vi "Get Package Filters.vi"(7 "LabVIEW Web Service Request":refnum<class "Web Request.lvclass">) -> ()   [LabVIEW 2016]
uses:
  <vilib>/wsapi/Web Request.lvclass
  Repo_class/Repo.lvclass/Repo.ctl
  Package_class/Package.lvclass/Package.ctl
  Repo_class/Read Packages.vi
  Package_class/Read RepoType.vi
  Package_class/Read RepoName.vi
  WSsupport/GV_Repos.vi
  <userlib>/_OpenG.lib/array/array.llb/Remove Duplicates from 1D Array (String)__ogtk.vi
  <vilib>/addons/JSON API/Variant JSON/Variant to JSON.vi
  Package_class/Package.lvclass
  WSsupport/WSsupport.lvlib
  Repo_class/Repo.lvclass
  <vilib>/addons/JSON API/Get Polymorphic/JSON GetSet.lvlib
  <vilib>/addons/JSON API/JSON Value/JSON Value.lvclass
  ServerErrors/ServerErrors.lvlib
  <vilib>/addons/JSON API/Variant JSON/Variant JSON.lvlib
panel:
  # "Use the Web Service Request input terminal to call the VIs on the Web Services palette. Do not remove it from the connector pane unless you don't need access to the palette."
  # "Each additional control wired to the connector pane will be available as an input in the URL. To include an indicator in terminal-mode output (the default setting), it must also be wired to the connector pane."
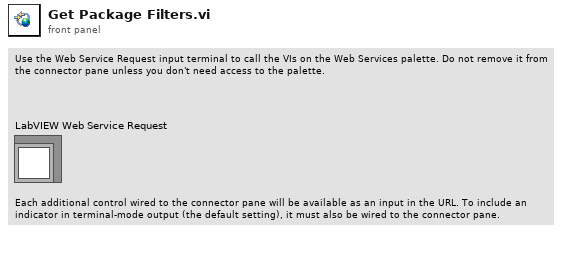
[diagram p1: front panel]
types:
  T1 = cluster{"RepoTypes":string[], "RepoNames":string[]}
  T2 = typedef "Packages.lvlib/Repo.lvclass/RepoType--enum.ctl" = enum16{"VIPM", "NIPM", "GPM"}
  T3 = typedef "ServerErrors.lvlib/Error Message--cluster.ctl" = cluster{"HTTP Code":i32, "JSON Response":cluster{"error":string, "reason":string}}
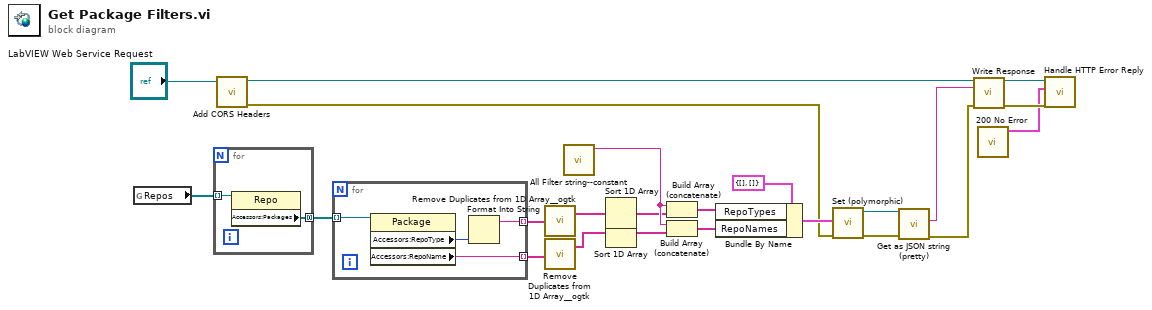
[diagram p0: block diagram]
diagram:
  n1 = global read "GV_Repos.vi" "Repos"() -> (w22:refnum<class "Repo.lvclass">[])
  n2 = for {
    tunnel: w22 -> [w25] mode=indexing
    tunnel: [w24] -> w21 mode=concatenating
    n3 = property class="Repo"(reference=w25) -> ("Accessors:Packages"=w24:refnum<class "Package.lvclass">[])  [unwired: 1 in, 2 out]
  }
  n4 = call "Add CORS Headers.vi"("LabVIEW Web Service Request"="LabVIEW Web Service Request") -> ("error out"=w12:errorcluster, "LabVIEW Web Service Request out"=w8:refnum<class "Web Request.lvclass">)  [unwired: 9 in]
  n5 = for {
    tunnel: w21 -> [w29] mode=indexing
    tunnel: [w27] -> w20 mode=indexing
    tunnel: [w26] -> w19 mode=indexing
    n6 = property class="Package"(reference=w29) -> ("Accessors:RepoType"=w28:T2, "Accessors:RepoName"=w26:string)  [unwired: 1 in, 2 out]
    n7 = Format Into String(w28) -> (resulting string=w27:string)  [unwired: 3 in, 1 out]
  }
  n8 = call-poly <userlib>:"Remove Duplicates from 1D Array__ogtk.vi"("Input Array"=w20) -> ("Output Array"=w17:string[])  [unwired: 1 out]
  n9 = call-poly <userlib>:"Remove Duplicates from 1D Array__ogtk.vi"("Input Array"=w19) -> ("Output Array"=w16:string[])  [unwired: 1 out]
  n10 = call "All Filter string--constant.vi"() -> ("All Filter string"=w3:string)  [unwired: 11 in]
  n11 = Sort 1D Array(array=w17) -> (sorted array=w2:string[])
  n12 = Sort 1D Array(array=w16) -> (sorted array=w1:string[])
  n13 = Build Array (concatenate)(w3, w2) -> (w4:string[])
  n14 = Build Array (concatenate)(w3, w1) -> (w5:string[])
  n15 = Bundle By Name(cluster=T1 {"RepoTypes"=[], "RepoNames"=[]}, "RepoTypes"=w4, "RepoNames"=w5) -> (w15:T1)
  n16 = call-poly <vilib>:"Set (polymorphic).vi"("error in (no error)"=w12, "Variant"=w15) -> ("error out"=w13:errorcluster, "JSON Value out"=w14:refnum<class "JSON Value.lvclass">)  [unwired: 8 in]
  n17 = call <vilib>:"Get as JSON string (pretty).vi"("error in (no error)"=w13, "JSON Value in"=w14) -> ("error out"=w6:errorcluster, "<JSON>"=w7:string)  [unwired: 8 in]
  n18 = call <vilib>:"Write Response.vi"("LabVIEW Web Service Request"=w8, "response string"=w7, "error in (no error)"=w6) -> ("LabVIEW Web Service Request out"=w11:refnum<class "Web Request.lvclass">, "error out"=w10:errorcluster)  [unwired: 11 in]
  n19 = call "200 No Error.vi"() -> ("no error"=w9:T3)  [unwired: 11 in]
  n20 = call "Handle HTTP Error Reply.vi"("error in (no error)"=w10, "HTTP Status Code"=w9, "Web Request in"=w11) -> ()  [unwired: 8 in, 1 out]
